vi "Get Network Endpoint Enqueuer.vi"(8 "error in":errorcluster, 11 "Study Actor in":refnum<class "Study Actor.lvclass">) -> (0 "error out":errorcluster, 1 "Connected":bool, 2 "Network Endpoint Enqueuer":refnum<class "Message Enqueuer.lvclass">, 3 "Study Actor out":refnum<class "Study Actor.lvclass">)   [LabVIEW 2023, in "Study Actor.lvlib" / "Study Actor.lvclass"]
uses:
  Study Actor.lvclass
  <vilib>/ActorFramework/Message Enqueuer/Message Enqueuer.lvclass
  Study Actor.lvclass/Study Actor.ctl
  <vilib>/Utility/error.llb/Error Cluster From Error Code.vi
  <vilib>/ErrorRing/Error Ring.xnode
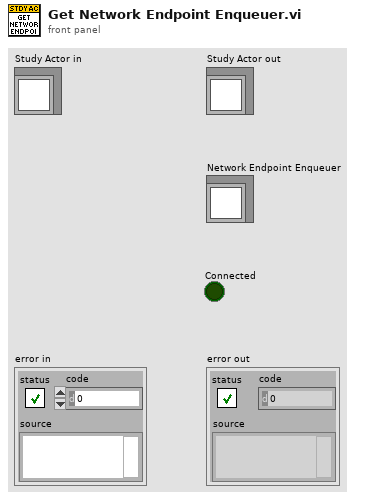
[diagram p1: front panel]
types:
  T1 = map{string, refnum<class "Message Enqueuer.lvclass">}
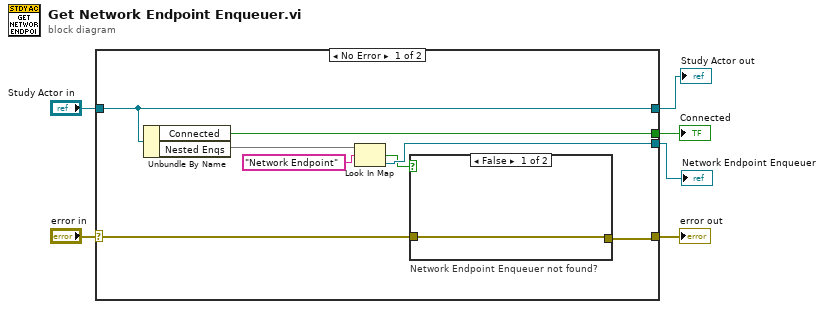
[diagram p0: block diagram]
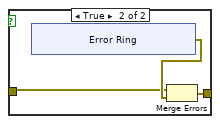
[diagram p2: hidden frame]
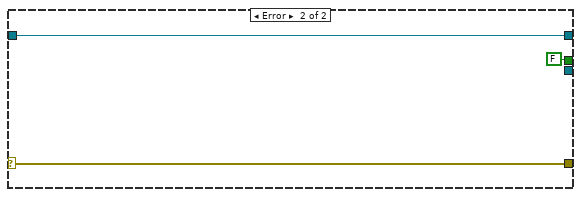
[diagram p3: hidden frame]
diagram:
  n1 = case shown="No Error" "error in" {
    selector: "error in" -> [w12 w26]
    tunnel: [w11 w26] -> w5
    tunnel: [w13 w25] -> w3
    tunnel: "Study Actor in" -> [w13 w25]
    tunnel: [w10 _] -> w2
    tunnel: [w7 FALSE ("Connected")] -> w1
    frame No Error {
      n2 = Unbundle By Name(w13) -> ("Connected"=w7:bool, "Nested Enqs"=w14:T1)
      n3 = Look In Map(map=w14, key="Network Endpoint") -> (key not found?=w8:bool, value=w10:refnum<class "Message Enqueuer.lvclass">)  [unwired: 1 in]
      n4 = case "Network Endpoint Enqueuer not found?" shown="False" w8 {
        tunnel: w12 -> [w15 w17]
        tunnel: [w15 w16] -> w11
        frame False {
        }
        frame True {
          n5 = xnode "Error Ring"() -> ("error out"=w18:errorcluster)
          n6 = Merge Errors(w17, w18) -> (w16:errorcluster)
        }
      }
    }
    frame Error {
    }
  }
  "error out" <- w5
  "Study Actor out" <- w3
  "Network Endpoint Enqueuer" <- w2
  "Connected" <- w1
